vi "TCP Data Stream (RT).vi"(0 "Data":dbl[][](array[numeric]), 5 "Error IN":errorcluster, 6 "Mode":T1) -> (16 "Connected?":bool, 19 "Error OUT":errorcluster)   [LabVIEW 2013]
uses:
  Controls/Stream TCP Data Stream Mode (RT).ctl
  Controls/Stream TCP Data Stream Mode.ctl
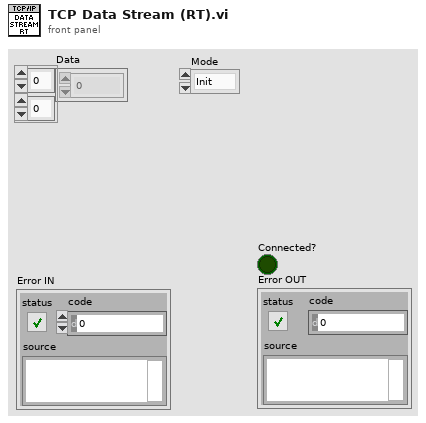
[diagram p1: front panel]
types:
  T1 = typedef "Stream TCP Data Stream Mode (RT).ctl" = enum16{"Init", "Write Data", "Close"}
  T2 = cluster{"Wait for HS":bool, "Connected?":bool, "Prev Data":dbl[][], "Time":dbl}
  T3 = typedef "Stream TCP Data Stream Mode.ctl" = enum16{"Init RT", "Init PC", "Connect RT", "Connect PC", "Write Data", "Read Data", "Close"}
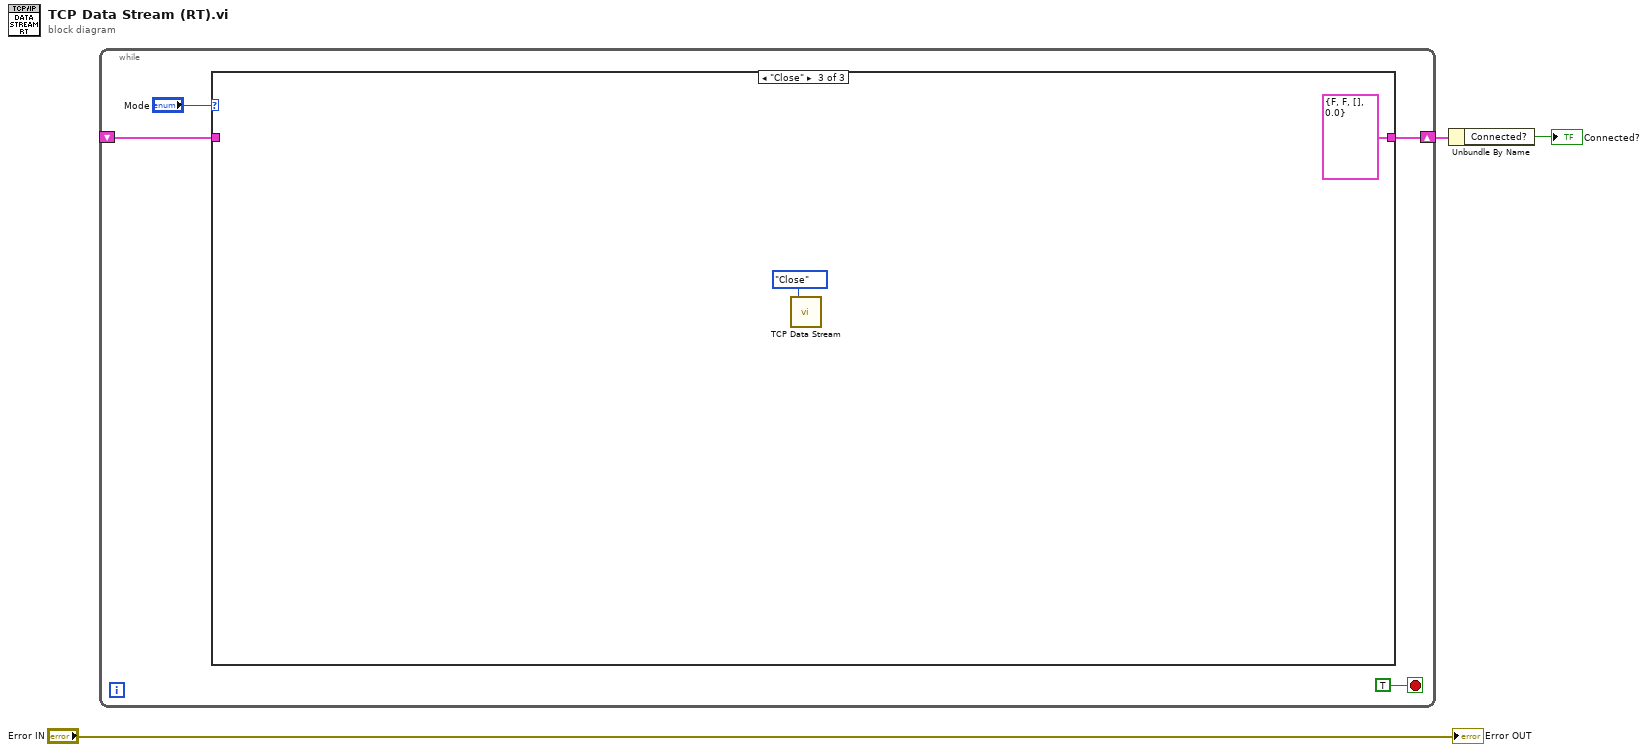
[diagram p0: block diagram]
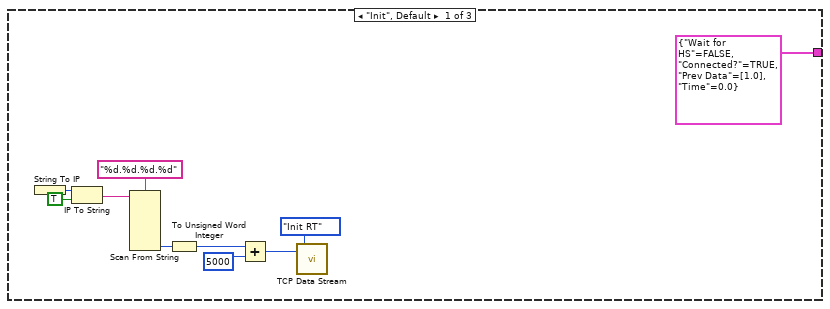
[diagram p2: hidden frame]
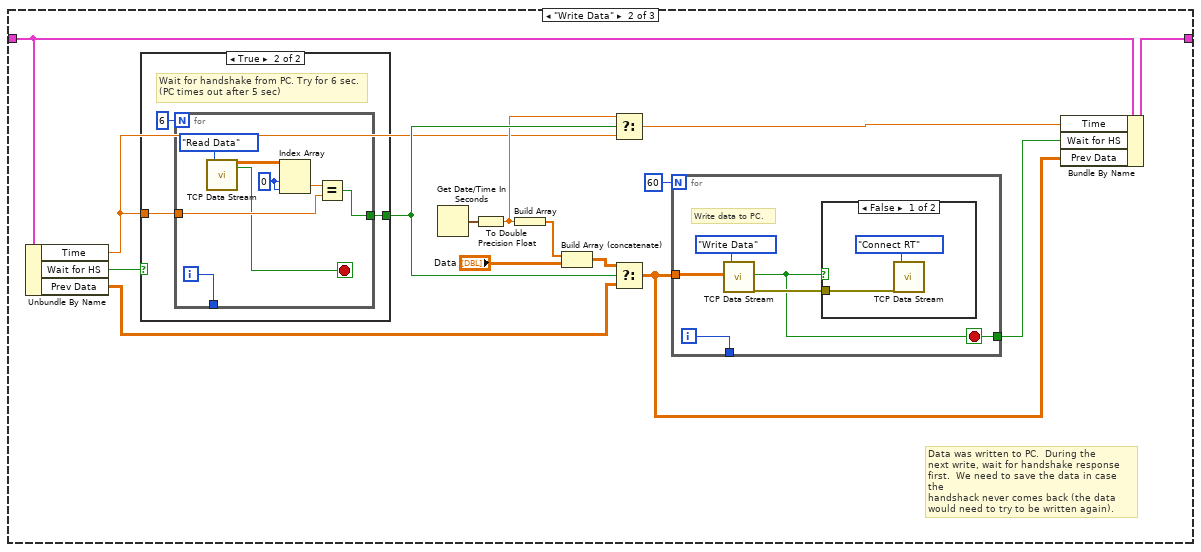
[diagram p3: hidden frame]
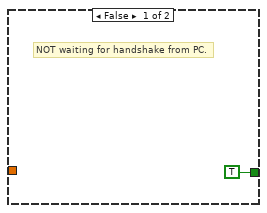
[diagram p5: hidden frame]
diagram:
  n1 = while {
    shift-right: [w5] -> w2
    shift-left: _ -> [w4]
    stop <- TRUE stop-if-true
    n2 = case shown="\"Close\"" "Mode" {
      tunnel: [T2 {"Wait for HS"=FALSE, "Connected?"=TRUE, "Prev Data"=[[1.0]], "Time"=0.0} w32 T2 {"Wait for HS"=FALSE, "Connected?"=FALSE, "Prev Data"=[], "Time"=0.0}] -> w5
      tunnel: w4 -> [_ w31 _]
      frame "Init", Default {
        n3 = String To IP() -> (0:w12:u32)  [unwired: 1 in]
        n4 = IP To String(1:TRUE ("dot notation? (F)"), 2:w12) -> (0:w10:string)
        n5 = Scan From String(format string="%d.%d.%d.%d", input string=w10) -> (output 4=w16:i32)  [unwired: 9 in, 3 out]
        n6 = To Unsigned Word Integer(number=w16) -> (unsigned 16bit integer=w14:u16)
        n7 = Add(x=w14, y=u16 5000 ("Port")) -> (x+y=w9:u16)
        n8 = call "TCP Data Stream.vi"("Port"=w9, "Mode"=Stream_TCP_Data_Stream_Mode."Init RT") -> ()  [unwired: 13 in, 5 out]
      }
      frame "Write Data" {
        # "Data was written to PC.  During the\nnext write, wait for handshake response\nfirst.  We need to save the data in case the\nhandshack never comes back (the data\nwould need to try to be written again)."
        n9 = Unbundle By Name(w31) -> ("Time"=w20:dbl, "Wait for HS"=w30:bool, "Prev Data"=w18:dbl[][])
        n10 = case shown="True" w30 {
          tunnel: [TRUE w42] -> w22
          tunnel: w20 -> [_ w41]
          frame False {
            # "NOT waiting for handshake from PC."
          }
          frame True {
            # "Wait for handshake from PC. Try for 6 sec.\n(PC times out after 5 sec)"
            n11 = for {
              N: 6 -> [_]
              tunnel: [w45] -> w42
              tunnel: w41 -> [w48]
              tunnel: [w46] -> _
              i -> [w46]
              stop <- w44 stop-if-true
              w49 = 0 ("index (row)")
              n12 = call "TCP Data Stream.vi"("Mode"=Stream_TCP_Data_Stream_Mode."Read Data") -> ("Data OUT"=w50:dbl[][], "New Data?"=w44:bool)  [unwired: 14 in, 3 out]
              n13 = Index Array(array=w50, index (row)=w49, index (col)=w49) -> (element=w47:dbl)
              n14 = Equal?(x=w47, y=w48) -> (x = y?=w45:bool)
            }
          }
        }
        n15 = Get Date/Time In Seconds() -> (seconds since 1Jan1904=w24:timestamp)
        n16 = To Double Precision Float(number=w24) -> (double precision float=w21:dbl)
        n17 = Build Array(w21) -> (w23:dbl[])
        n18 = Build Array (concatenate)(w23, "Data") -> (w25:dbl[][])
        n19 = Select(t=w21, s=w22, f=w20) -> (s? t:f=w19:dbl)
        n20 = Select(t=w25, s=w22, f=w18) -> (s? t:f=w29:dbl[][])
        n21 = for {
          N: 60 -> [_]
          tunnel: w29 -> [w36]
          tunnel: [w34] -> _
          tunnel: [w33] -> w27
          i -> [w34]
          stop <- w33 stop-if-true
          # "Write data to PC."
          n22 = call "TCP Data Stream.vi"("Data IN"=w36, "Mode"=Stream_TCP_Data_Stream_Mode."Write Data") -> ("Connected?"=w33:bool, "Error OUT"=w35:errorcluster)  [unwired: 13 in, 3 out]
          n23 = case shown="False" w33 {
            tunnel: w35 -> [w38 _]
            frame False {
              n24 = call "TCP Data Stream.vi"("Error IN"=w38, "Mode"=Stream_TCP_Data_Stream_Mode."Connect RT") -> ()  [unwired: 13 in, 5 out]
            }
            frame True {
            }
          }
        }
        n25 = Bundle By Name(cluster=w31, "Time"=w19, "Wait for HS"=w27, "Prev Data"=w29) -> (w32:T2)
      }
      frame "Close" {
        n26 = call "TCP Data Stream.vi"("Mode"=Stream_TCP_Data_Stream_Mode."Close") -> ()  [unwired: 14 in, 5 out]
      }
    }
  }
  n27 = Unbundle By Name(w2) -> ("Connected?"=→"Connected?":bool)
  "Error OUT" <- "Error IN"
